vi "ITX to TDMS.vi"(8 "error in (no error)":errorcluster, 10 "file (use dialog)":path=path "P:/sample/GaAs/GaAs quantum dots/2008/PL Map/A1 735/060731ASBA_A1_6.0.itx", 11 "LVtoITX in":refnum<class "LVtoITX.lvclass">) -> (0 "error out":errorcluster, 3 "LVtoITX out":refnum<class "LVtoITX.lvclass">)   [LabVIEW 2016, in "LVtoITX.lvclass"]
uses:
  LVtoITX.lvclass
  LVtoITX.lvclass/LVtoITX.ctl
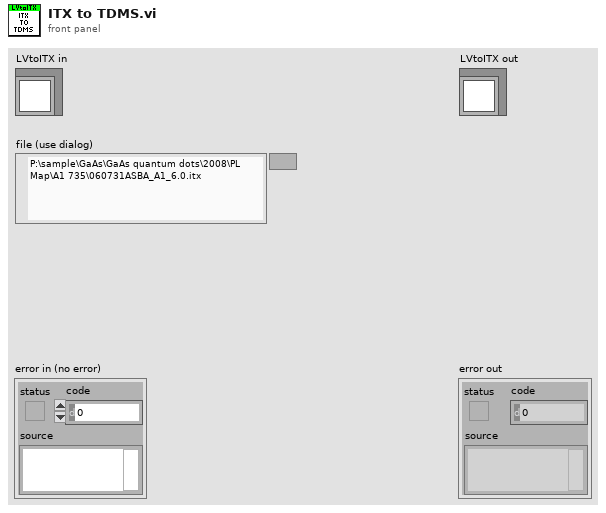
[diagram p1: front panel]
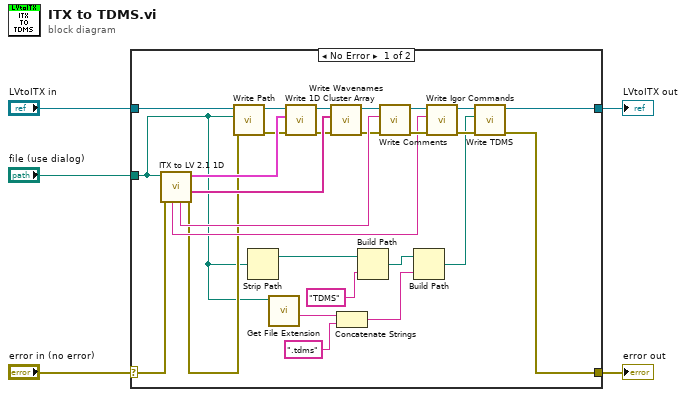
[diagram p0: block diagram]
diagram:
  n1 = case shown="No Error" "error in (no error)" {
    selector: "error in (no error)" -> [w32 w34]
    tunnel: [w15 w34] -> w4
    tunnel: [w14 w33] -> w2
    tunnel: "LVtoITX in" -> [w30 w33]
    tunnel: "file (use dialog)" -> [w11 _]
    frame No Error {
      n2 = call "ITX to LV 2.1 1D.vi"("error in"=w32, "file (use dialog)"=w11) -> ("error out"=w16:errorcluster, "base wavenames"=w29:string[], "1D Cluster Array"=w28:cluster{"array type (2D Dbl)":dbl[]}[], "Notes"=w31:string, "Commands"=w19:string)  [unwired: 4 in, 1 out]
      n3 = call "Write Path.vi"("error in (no error)"=w16, "Path"=w11, "LVtoITX in"=w30) -> ("error out"=w26:errorcluster, "LVtoITX out"=w27:refnum<class "LVtoITX.lvclass">)  [unwired: 7 in]
      n4 = Strip Path(path=w11) -> (stripped path=w6:path)  [unwired: 1 out]
      n5 = call <vilib>:"Get File Extension.vi"("file"=w11) -> ("filename without extension"=w13:string)  [unwired: 6 in, 4 out]
      n6 = call "Write 1D Cluster Array.vi"("error in (no error)"=w26, "1D Cluster Array"=w28, "LVtoITX in"=w27) -> ("error out"=w24:errorcluster, "LVtoITX out"=w25:refnum<class "LVtoITX.lvclass">)  [unwired: 7 in]
      n7 = call "Write Wavenames.vi"("error in (no error)"=w24, "Wavenames"=w29, "LVtoITX in"=w25) -> ("error out"=w22:errorcluster, "LVtoITX out"=w23:refnum<class "LVtoITX.lvclass">)  [unwired: 7 in]
      n8 = Concatenate Strings(w13, ".tdms" ("string")) -> (w12:string)
      n9 = Build Path(base path=w6, name or relative path="TDMS" ("string")) -> (appended path=w7:path)
      n10 = call "Write Comments.vi"("error in (no error)"=w22, "Comments"=w31, "LVtoITX in"=w23) -> ("error out"=w20:errorcluster, "LVtoITX out"=w21:refnum<class "LVtoITX.lvclass">)  [unwired: 7 in]
      n11 = Build Path(base path=w7, name or relative path=w12) -> (appended path=w10:path)
      n12 = call "Write Igor Commands.vi"("error in (no error)"=w20, "Igor Commands"=w19, "LVtoITX in"=w21) -> ("error out"=w17:errorcluster, "LVtoITX out"=w18:refnum<class "LVtoITX.lvclass">)  [unwired: 7 in]
      n13 = call "Write TDMS.vi"("error in (no error)"=w17, "path"=w10, "LVtoITX in"=w18) -> ("error out"=w15:errorcluster, "LVtoITX out"=w14:refnum<class "LVtoITX.lvclass">)  [unwired: 7 in]
    }
    frame Error {
    }
  }
  "error out" <- w4
  "LVtoITX out" <- w2
